vi "CreateSBDSavePath.vi"(9 "Base Save Path":path, 10 "Month":string, 11 "Day":string) -> (3 "File Path Control":path)   [LabVIEW 2014]
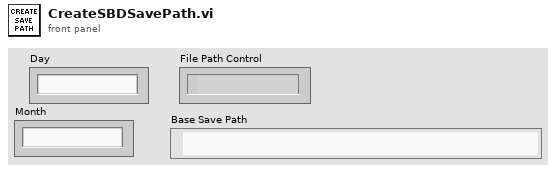
[diagram p1: front panel]
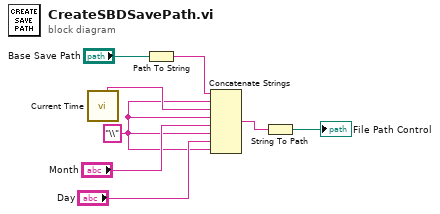
[diagram p0: block diagram]
diagram:
  w1 = "\\" ("string")
  n1 = call "Current Time.vi"() -> ("Year"=w5:string)  [unwired: 6 in, 5 out]
  n2 = Path To String(path="Base Save Path") -> (string=w2:string)
  n3 = Concatenate Strings(w2, w1, w5, w1, "Month", w1, "Day", w1) -> (w6:string)
  n4 = String To Path(string=w6) -> (path=→"File Path Control":path)
